vi "set name.vi"(8 "error in (no error)":errorcluster caption="에러 입력(에러 없음)", 11 "Waveform Gen 입력":refnum<class "Waveform Gen.lvclass">) -> (0 "error out":errorcluster caption="에러 출력", 3 "Waveform Gen 출력":refnum<class "Waveform Gen.lvclass">)   [LabVIEW 2020, in "Waveform Gen.lvclass"]
uses:
  Waveform Gen.lvclass
  Waveform Gen.lvclass/Waveform Gen.ctl
  Waveform Obj/Waveform Obj.lvclass/Waveform Obj.ctl
  Accessors/Read frequency.vi
  Accessors/Read cycle.vi
  Accessors/Read scale.vi
  Waveform Obj/Accessors/Write name.vi
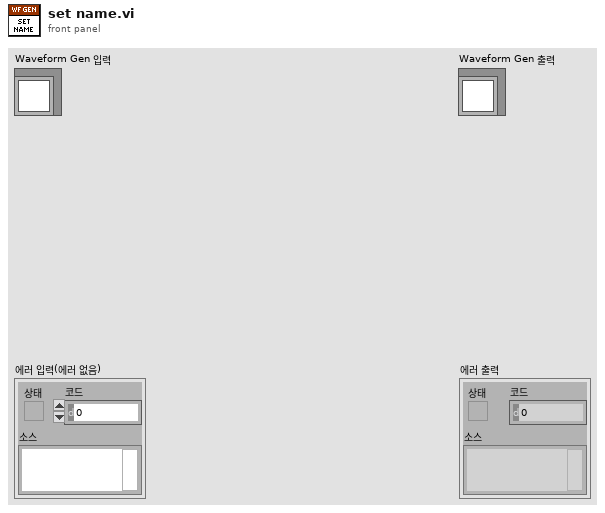
[diagram p1: front panel]
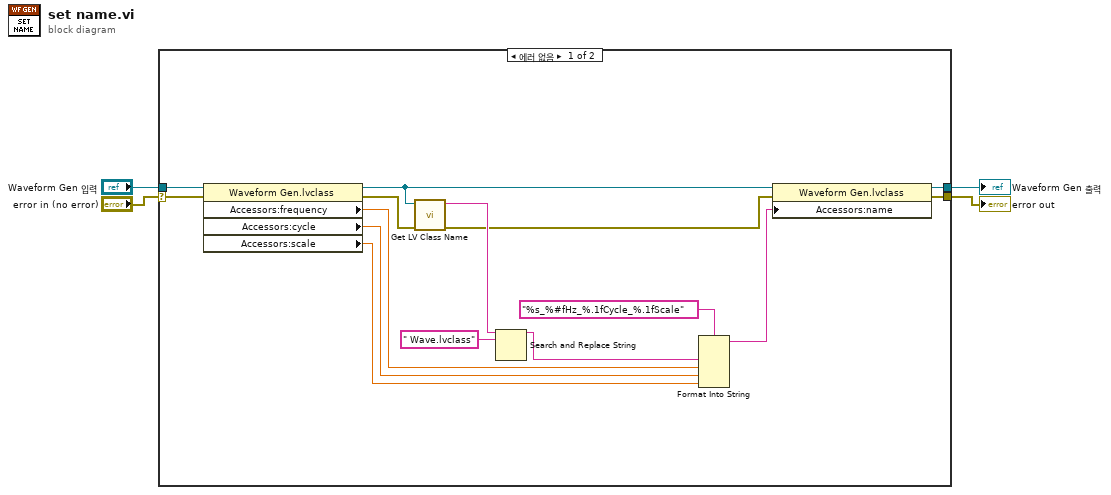
[diagram p0: block diagram]
diagram:
  n1 = case shown="에러 없음" "error in (no error)" {
    selector: "error in (no error)" -> [w15 w20]
    tunnel: "Waveform Gen 입력" -> [w14 w21]
    tunnel: [w12 w20] -> w2
    tunnel: [w11 w21] -> w1
    frame No Error {
      n2 = property class="Waveform Gen.lvclass"(reference=w14, error in=w15) -> (reference out=w10:refnum<class "Waveform Gen.lvclass">, error out=w13:errorcluster, "Accessors:frequency"=w18:dbl, "Accessors:cycle"=w17:dbl, "Accessors:scale"=w16:dbl)
      n3 = call <vilib>:"Get LV Class Name.vi"("error in (no error)"=w13, "object"=w10) -> ("error out"=w8:errorcluster, "class name"=w9:string)  [unwired: 8 in]
      n4 = Search and Replace String(input string=w9, search string=" Wave.lvclass" ("검색 문자열")) -> (result string=w5:string)  [unwired: 6 in, 3 out]
      n5 = Format Into String(format string="%s_%#fHz_%.1fCycle_%.1fScale" ("포맷 문자열"), w5, w18, w17, w16) -> (resulting string=w7:string)  [unwired: 2 in, 1 out]
      n6 = property class="Waveform Gen.lvclass"(reference=w10, error in=w8, "Accessors:name"=w7) -> (reference out=w11:refnum<class "Waveform Gen.lvclass">, error out=w12:errorcluster)
    }
    frame Error {
    }
  }
  "error out" <- w2
  "Waveform Gen 출력" <- w1
